vi "Rate Scan. Ajuste por minimos cuadrados.vi"(4 "V asic Theorical":dbl[](array[numeric]), 5 "V asic Real":dbl[](array[numeric]), 6 "Salida B":dbl[][][](array[numeric]), 7 "Salida A":dbl[][][](array[numeric])) -> (0 "Salida B rectificada":dbl[][][](array[numeric]), 1 "Cruze por 0 Salida B":dbl[][](array[numeric]), 2 "Cruze por 0 Salida A":dbl[][](array[numeric]), 3 "Salida A rectificada":dbl[][][](array[numeric]))   [LabVIEW 2019]
uses:
  <vilib>/Analysis/6fits.llb/Curve Fitting Criteria.ctl
  <vilib>/Analysis/NI_AALPro.lvlib
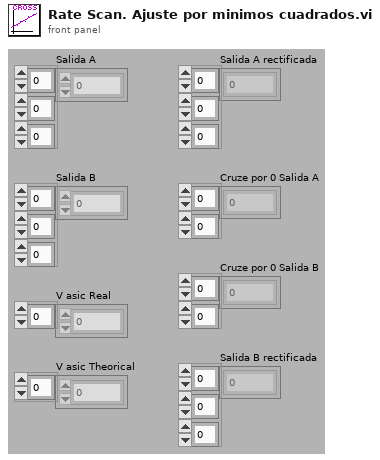
[diagram p1: front panel]
types:
  T1 = typedef "NI_AALPro.lvlib/Curve Fitting Criteria.ctl" = u16
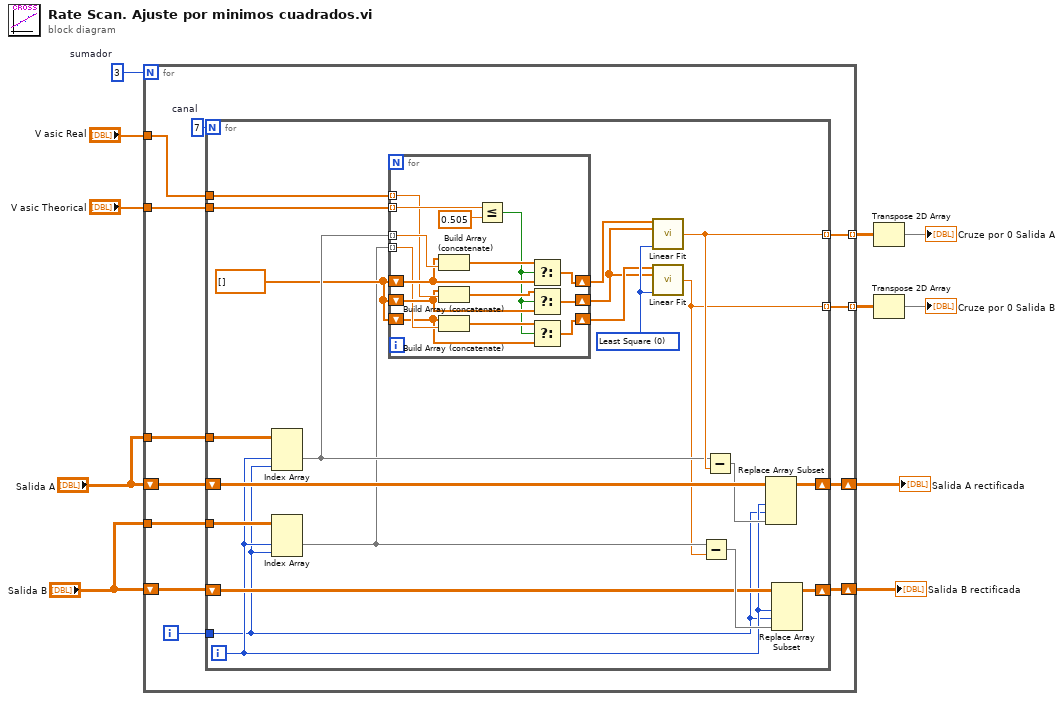
[diagram p0: block diagram]
diagram:
  w2 = 3  # sumador
  n1 = for {
    N: w2 -> [_]
    tunnel: "Salida A" -> [w23]
    tunnel: "V asic Real" -> [w20]
    tunnel: [w19] -> w4 mode=indexing
    tunnel: "V asic Theorical" -> [w18]
    shift-right: [w16] -> w10
    shift-left: "Salida A" -> [w17]
    tunnel: "Salida B" -> [w15]
    shift-right: [w13] -> w11
    shift-left: "Salida B" -> [w14]
    tunnel: [w12] -> w9 mode=indexing
    i -> [w22]
    w21 = 7  # canal
    n2 = for {
      N: w21 -> [_]
      tunnel: w23 -> [w44]
      tunnel: w22 -> [w26]
      tunnel: w20 -> [w42]
      tunnel: [w43] -> w19 mode=indexing
      tunnel: w18 -> [w40]
      shift-right: [w36] -> w16
      shift-left: w17 -> [w38]
      tunnel: w15 -> [w35]
      shift-right: [w25] -> w13
      shift-left: w14 -> [w29]
      tunnel: [w24] -> w12 mode=indexing
      i -> [w27]
      w34 = dbl[] []
      w32 = T1 0 items=["Least Square", "Least Absolute Residual", "Bisquare"] ("method")
      n3 = Index Array(array=w44, index (dim 1)=w27, index (dim 2)=w26) -> (element=w41:dbl[])  [unwired: 1 in]
      n4 = Index Array(array=w35, index (dim 1)=w27, index (dim 2)=w26) -> (element=w28:dbl[])  [unwired: 1 in]
      n5 = for {
        tunnel: w42 -> [w54] mode=indexing
        tunnel: w41 -> [w57] mode=indexing
        tunnel: w40 -> [w59] mode=indexing
        shift-right: [w50] -> w39
        shift-left: w34 -> [w55]
        shift-right: [w51] -> w30
        shift-left: w34 -> [w52]
        shift-right: [w45] -> w31
        shift-left: w34 -> [w47]
        tunnel: w28 -> [w49] mode=indexing
        n6 = Build Array (concatenate)(w55, w57) -> (w56:dbl[])
        n7 = Build Array (concatenate)(w52, w54) -> (w53:dbl[])
        n8 = Build Array (concatenate)(w47, w49) -> (w48:dbl[])
        n9 = Less Or Equal?(x=w59, y=0.505) -> (x <= y?=w46:bool)
        n10 = Select(t=w56, s=w46, f=w55) -> (s? t:f=w50:dbl[])
        n11 = Select(t=w53, s=w46, f=w52) -> (s? t:f=w51:dbl[])
        n12 = Select(t=w48, s=w46, f=w47) -> (s? t:f=w45:dbl[])
      }
      n13 = call <vilib>:"Linear Fit.vi"("Y"=w39, "X"=w30, "method"=w32) -> ("intercept"=w43:dbl)  [unwired: 8 in, 4 out]
      n14 = call <vilib>:"Linear Fit.vi"("Y"=w31, "X"=w30, "method"=w32) -> ("intercept"=w24:dbl)  [unwired: 8 in, 4 out]
      n15 = Subtract(x=w28, y=w24) -> (x-y=w33:dbl[])
      n16 = Subtract(x=w41, y=w43) -> (x-y=w37:dbl[])
      n17 = Replace Array Subset(array=w38, new element=w37, index (dim 1)=w27, index (dim 2)=w26) -> (w36:dbl[][][])  [unwired: 1 in]
      n18 = Replace Array Subset(array=w29, new element=w33, index (dim 1)=w27, index (dim 2)=w26) -> (w25:dbl[][][])  [unwired: 1 in]
    }
  }
  "Salida B rectificada" <- w11
  "Salida A rectificada" <- w10
  n19 = Transpose 2D Array(2D array=w4) -> (transposed array=→"Cruze por 0 Salida A":dbl[][])
  n20 = Transpose 2D Array(2D array=w9) -> (transposed array=→"Cruze por 0 Salida B":dbl[][])
